vi "Execute.vi"(8 "error in (no error)":errorcluster, 10 "Motor in":refnum<class "Motor.lvclass">, 11 "Wait in":refnum<class "Home.lvclass">) -> (0 "error out":errorcluster, 1 "Status message":string, 2 "Motor out":refnum<class "Motor.lvclass">, 3 "Wait out":refnum<class "Home.lvclass">)   [LabVIEW 2013, in "PowderDeposition.lvlib" / "Home.lvclass"]
uses:
  Home.lvclass
  Motor/Motor.lvclass
  Home.lvclass/Home.ctl
  Move-Absolute/Move-Absolute.lvclass
  Move-Absolute/Move-Absolute-settings.ctl
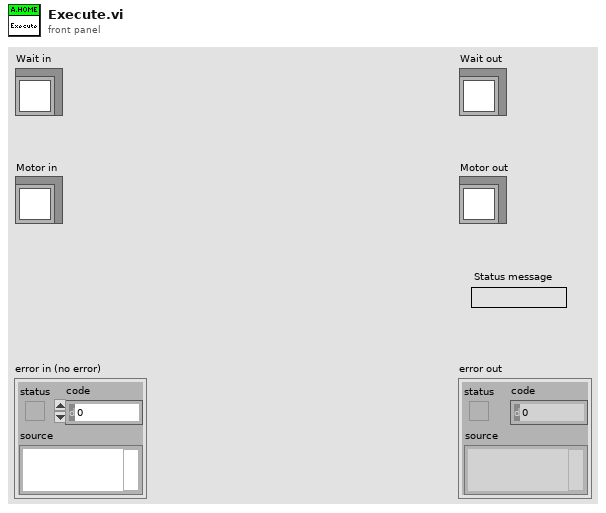
[diagram p1: front panel]
types:
  T1 = typedef "PowderDeposition.lvlib/Move-Absolute.lvclass/Move-Absolute-settings.ctl" = cluster{"Position":dbl, "Speed":dbl, "Min duration":dbl}
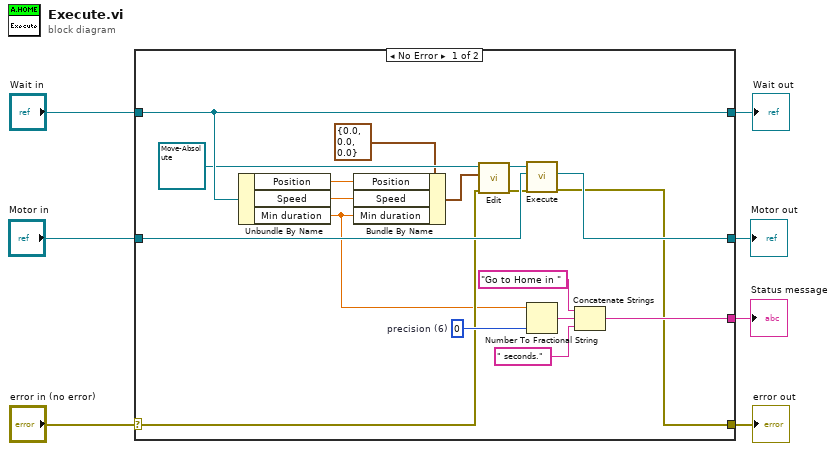
[diagram p0: block diagram]
diagram:
  n1 = case shown="No Error" "error in (no error)" {
    selector: "error in (no error)" -> [w10 w28]
    tunnel: [w9 w28] -> w6
    tunnel: [w25 w27] -> w4
    tunnel: "Wait in" -> [w25 w27]
    tunnel: [w21 _] -> w3
    tunnel: "Motor in" -> [w13 w26]
    tunnel: [w12 w26] -> w1
    frame No Error {
      w20 = i16 0  # precision (6)
      n2 = Unbundle By Name(w25) -> ("Position"=w17:dbl, "Speed"=w16:dbl, "Min duration"=w8:dbl)
      n3 = Bundle By Name(cluster=T1 {"Position"=0.0, "Speed"=0.0, "Min duration"=0.0} ("Edit dialog"), "Position"=w17, "Speed"=w16, "Min duration"=w8) -> (w15:T1)
      n4 = call-dynamic "Edit.vi"("error in (no error)"=w10, "Edit dialog"=w15, "Action in"=refnum<class "Move-Absolute.lvclass"> refnum ("Move-Absolute.lvclass")) -> ("error out"=w11:errorcluster, "Action out"=w14:refnum<class "Move-Absolute.lvclass">)  [unwired: 7 in]
      n5 = call-dynamic "Execute.vi"("error in (no error)"=w11, "Motor in"=w13, "Move in"=w14) -> ("error out"=w9:errorcluster, "Motor out"=w12:refnum<class "Motor.lvclass">)  [unwired: 5 in, 2 out]
      n6 = Number To Fractional String(number=w8, precision (6)=w20) -> (F-format string=w24:string)  [unwired: 2 in]
      n7 = Concatenate Strings("Go to Home in ", w24, " seconds.") -> (w21:string)
    }
    frame Error {
    }
  }
  "error out" <- w6
  "Wait out" <- w4
  "Status message" <- w3
  "Motor out" <- w1
